vi "regser Main.vi"() -> ()   [LabVIEW 2015]
doc: "This template is for the Queued Message Handler design pattern.\n\nThe Event Handling Loop generates messages based on user interface actions.\n\nThe Message Handling Loop processes messages generated by the Event Handling Loop, or by other messages. The messages are string values, so new messages can be added easily to the Message Cases case structure in the Message Handling Loop. Each message cluster can also provide an optional value for Message Data, which is a variant that can be converted to whatever message-specific data is required."
uses:
  Type Definitions/status_LED.ctl
  controls/regser UI Data.ctl
  init_config/typedef/init_config_data.ctl
  controls/config Data.ctl
  support/Message Queue/Enqueue Message (Single).vi
  <vilib>/Utility/error.llb/Error Cluster From Error Code.vi
  <vilib>/ErrorRing/Error Ring.xnode
  support/Message Queue/regser Message Queue.lvlib
  support/User Event - Stop/regser User Event - Stop.lvlib
panel:
  out "sw ver":string
  out "Enpoint":string
  in  "Exit Button":bool
  out "Target":dbl caption="Tgt"
  out "No. rej":i32
  out "Rejected":i32(slide) caption="Rejected test logs" scale=0.0..20.0
  out "No. pend":i32
  out "Pending":i32(slide) caption="Pending test logs" scale=0.0..20.0
  out "No. acc":i32
  out "Accepted":i32(slide) caption="Accepted test logs" scale=0.0..1000.0
  out "ext.":string caption="searching for"
  in  "Stop Button":bool
  in  "Start Button":bool
  out "Messages":string
  out "status":T1
  out "Elapsed time":dbl format="%.1f"
  out "Run":bool
  out "Display <Replace Me>":string
  # "QMH based"
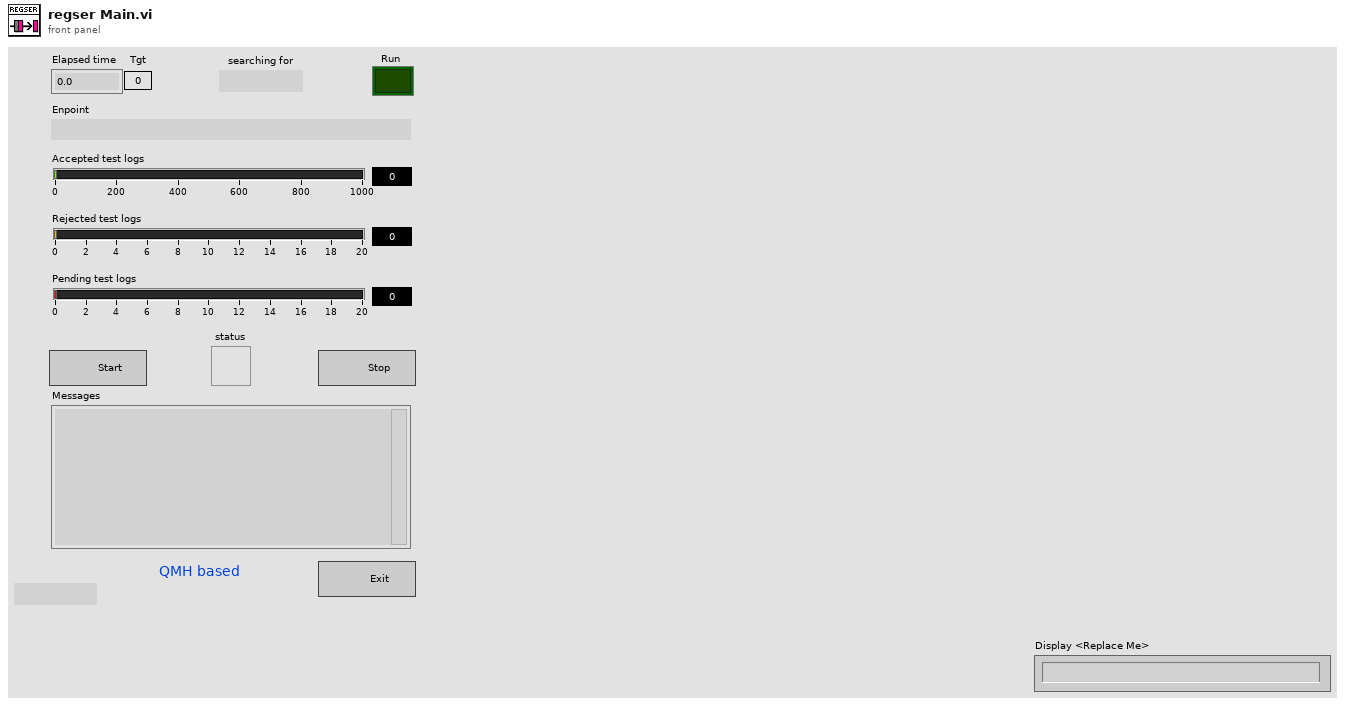
[diagram p1: front panel]
types:
  T1 = typedef "status_LED.ctl" = bool
  T2 = typedef "config Data.ctl" = cluster{"Boolean <Replace Me>":bool, "String <Replace Me>":string, "Numeric <Replace Me>":dbl, "http timeout":cluster{"get_timeout":i32, "post_timeout":i32}}
  T3 = typedef "regser UI Data.ctl" = cluster{"Boolean <Replace Me>":bool, "String <Replace Me>":string, "Numeric <Replace Me>":dbl, "Do Something Ref":refnum<vi>, "Do Something Else Ref":refnum<vi>, "Data Display Ref":refnum<vi>, "Exit Button Ref":refnum<vi>, "Cfg Data":T4, "Folder Path out":path, "All Files in Dir":path[], "No. of Files":i32, "Err Msg":string, "Err status":bool}
  T4 = typedef "init_config_data.ctl" = cluster{"http timeout":cluster{"get_timeout":i32, "post_timeout":i32}, "folders":cluster{"test_log_base_path":string, "accepted_folder_name":string, "rejected_folder_name":string}, "end_point":string, "file_ext":string, "holding time":dbl}
  T5 = typedef "regser Message Queue.lvlib/All Message Queues.ctl" = cluster{"UI":refnum<queue>, "CNFG":refnum<queue>}
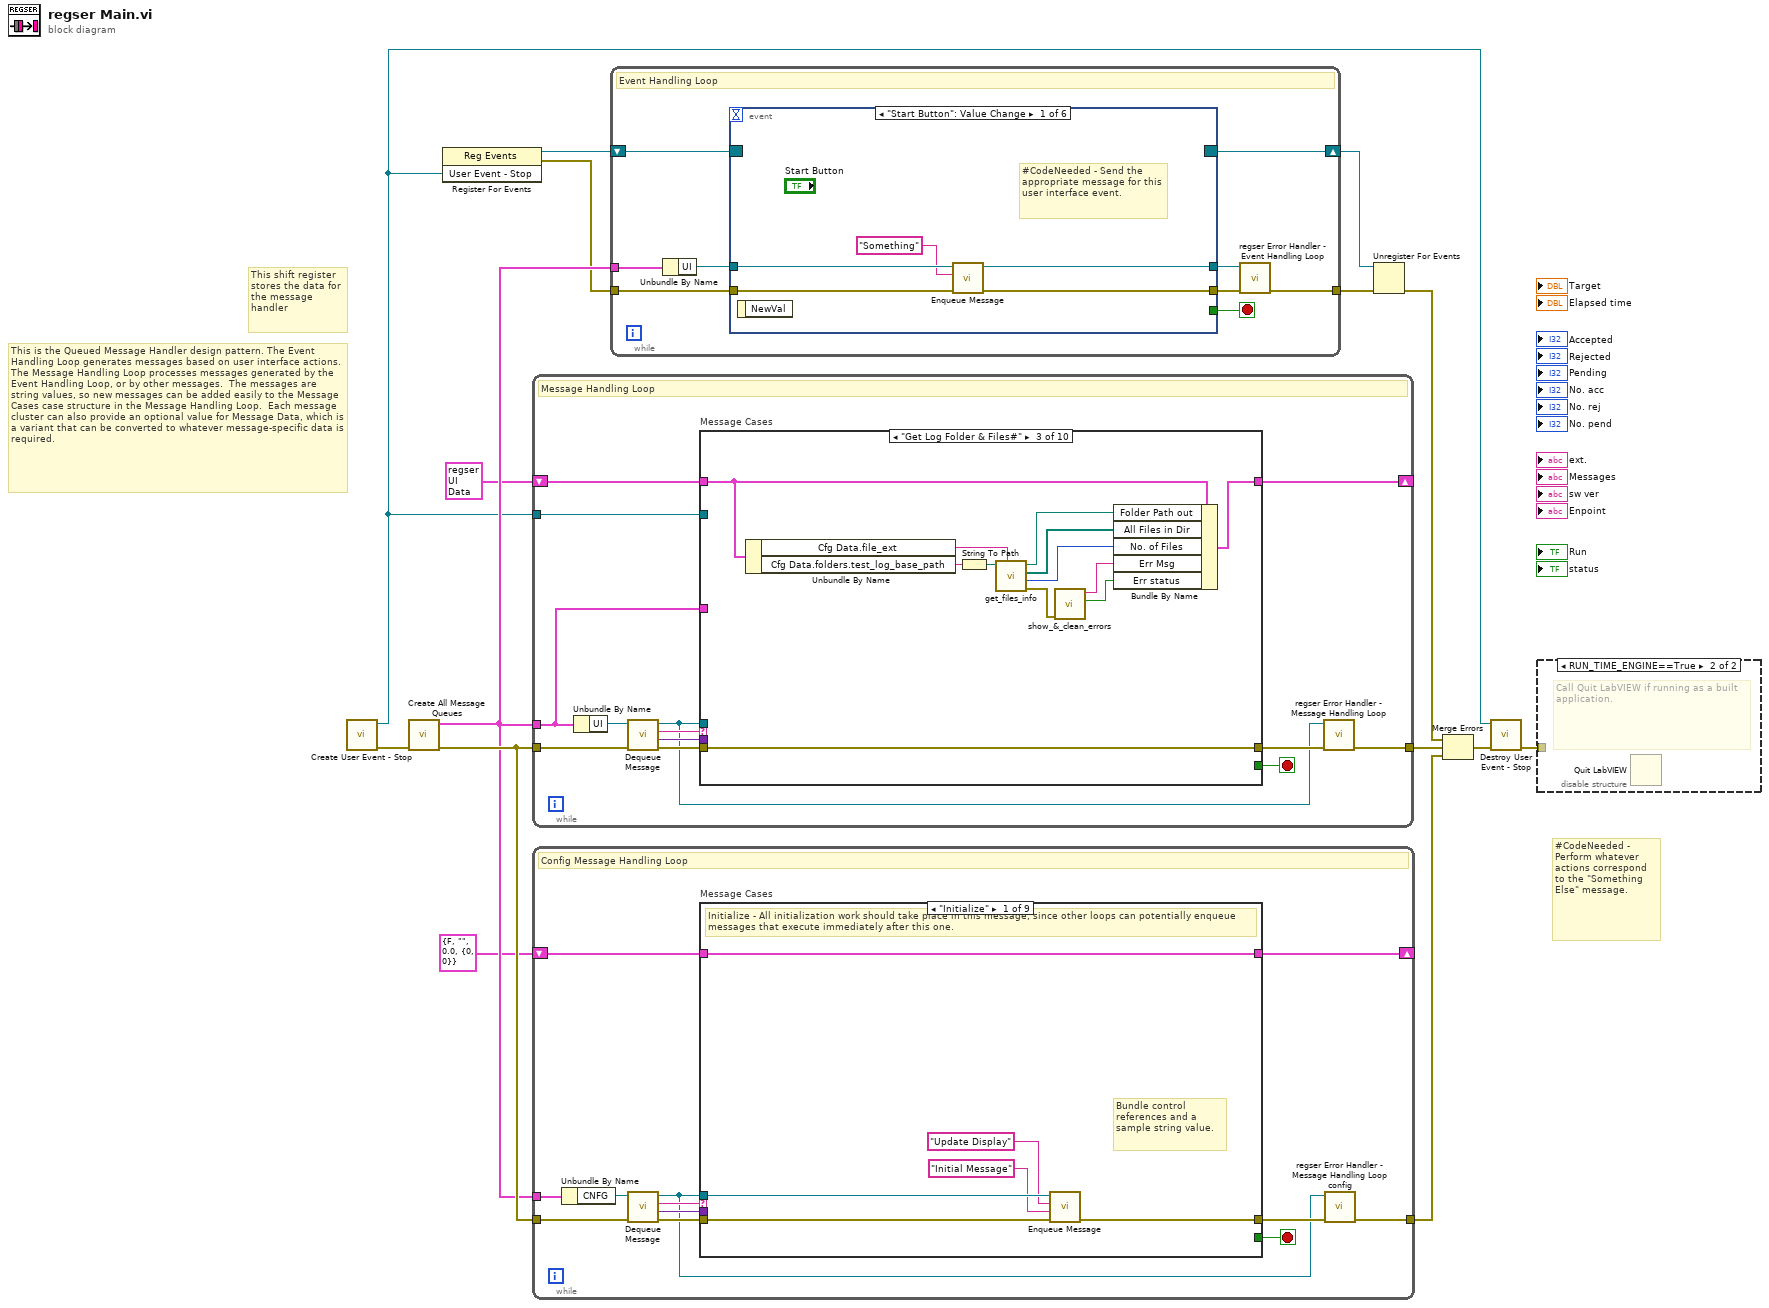
[diagram p0: block diagram]
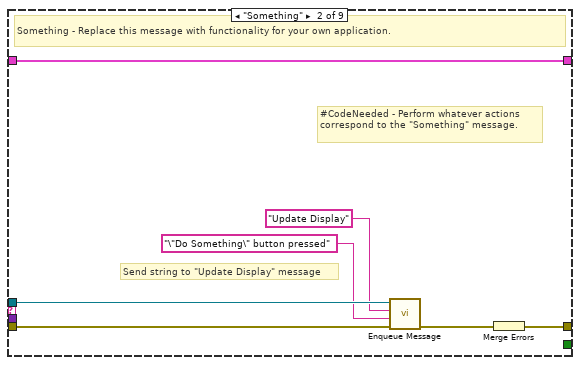
[diagram p2: hidden frame]
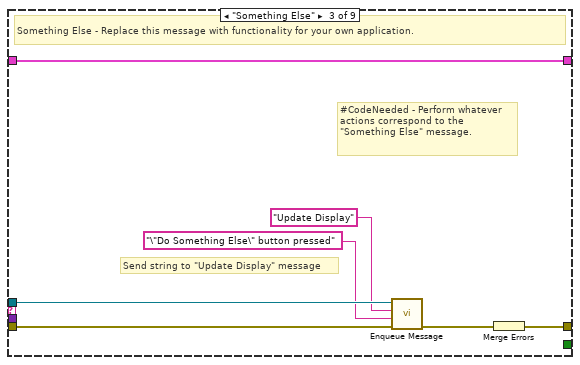
[diagram p3: hidden frame]
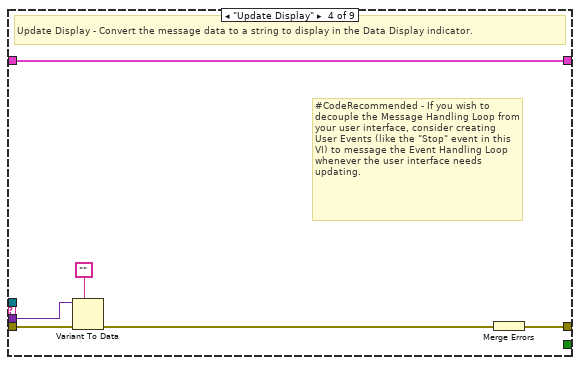
[diagram p4: hidden frame]
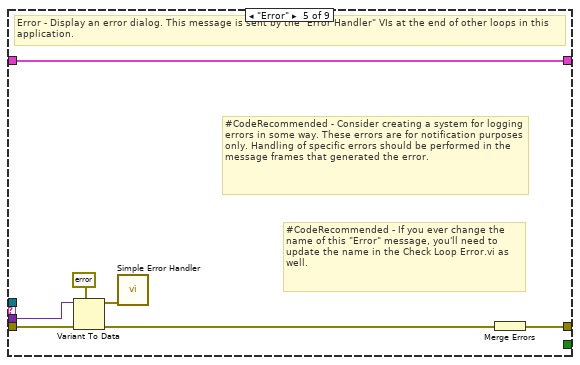
[diagram p5: hidden frame]
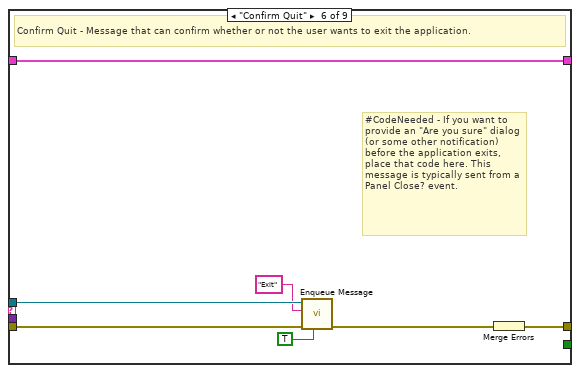
[diagram p6: hidden frame]
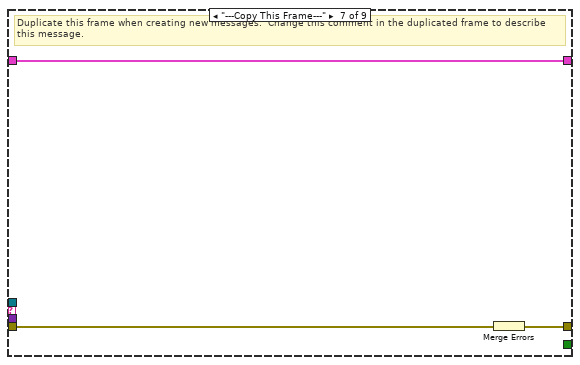
[diagram p7: hidden frame]
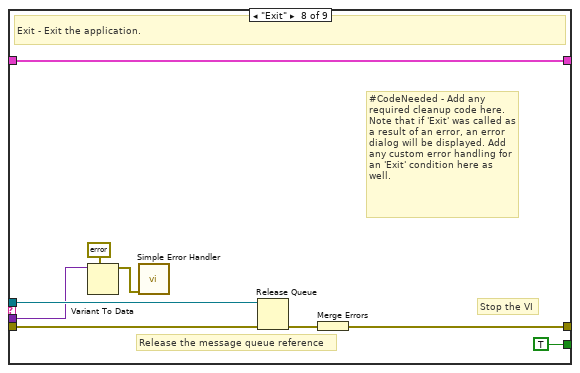
[diagram p8: hidden frame]
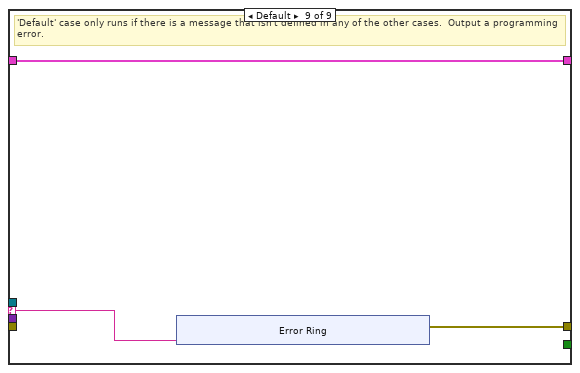
[diagram p9: hidden frame]
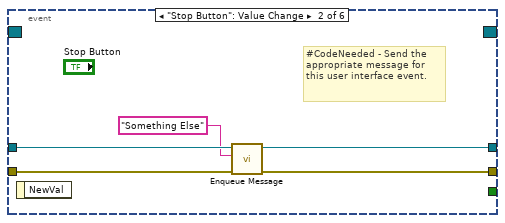
[diagram p11: hidden frame]
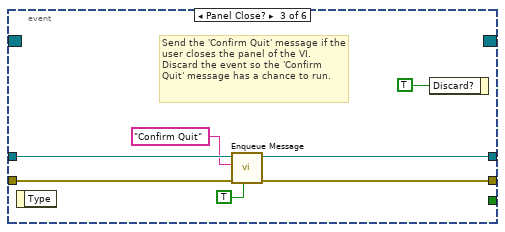
[diagram p12: hidden frame]
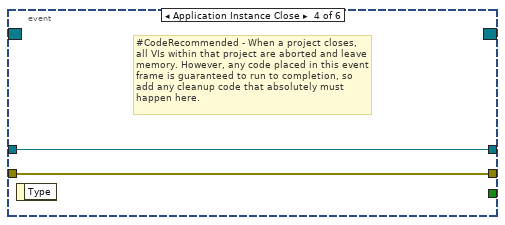
[diagram p13: hidden frame]
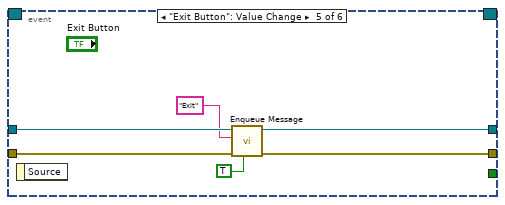
[diagram p14: hidden frame]
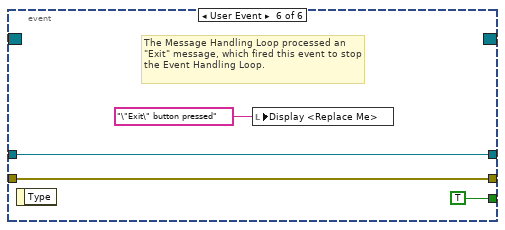
[diagram p15: hidden frame]
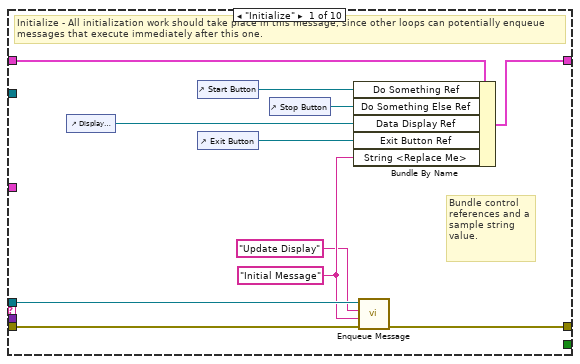
[diagram p16: hidden frame]
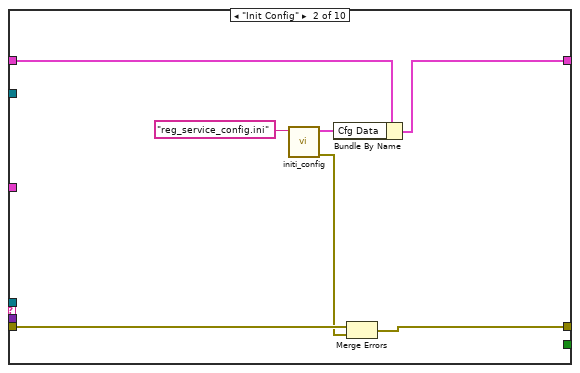
[diagram p17: hidden frame]
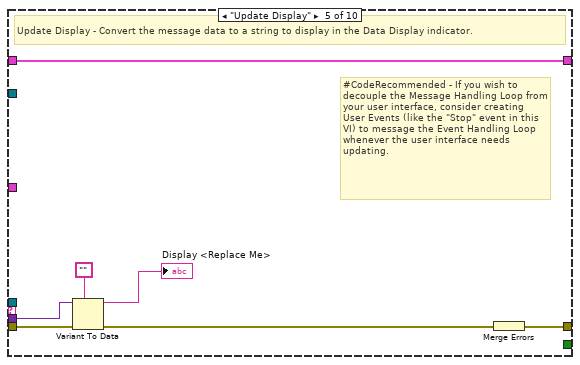
[diagram p19: hidden frame]
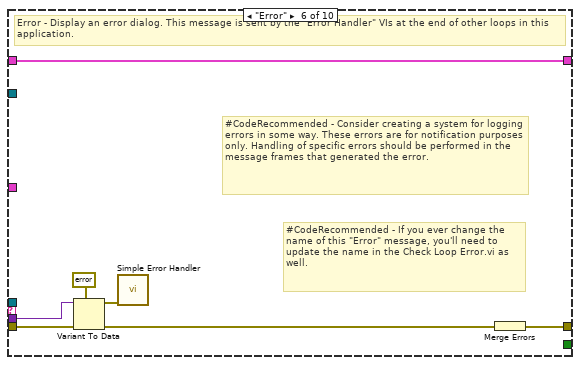
[diagram p20: hidden frame]
diagram:
  # "#CodeNeeded - Perform whatever actions correspond to the \"Something Else\" message."
  # "This is the Queued Message Handler design pattern. The Event Handling Loop generates messages based on user interface actions. The Message Handling Loop processes messages generated by the Event Handling Loop, or by other messages.  The messages are string values, so new messages can be added easily to the Message Cases case structure in the Message Handling Loop.  Each message cluster can also provide an optional value for Message Data, which is a variant that can be converted to whatever message-specific data is required."
  # "This shift register stores the data for the message handler"
  n1 = call "Create User Event - Stop.vi"() -> ("error out"=w12:errorcluster, "User Event - Stop"=w4:refnum<user-event>)  [unwired: 10 in]
  n2 = call "Create All Message Queues.vi"("error in (no error)"=w12) -> ("error out"=w15:errorcluster, "Message Queues out"=w14:T5)  [unwired: 9 in]
  n3 = register-events(w4) -> (reference out=w5:refnum<event-registration>, error out=w1:errorcluster)  [unwired: 2 in]
  n4 = while {
    shift-right: [w27] -> _
    shift-left: T3 {"Boolean <Replace Me>"=FALSE, "String <Replace Me>"="", "Numeric <Replace Me>"=0.0, "Do Something Ref"=refnum, "Do Something Else Ref"=refnum, "Data Display Ref"=refnum, "Exit Button Ref"=refnum, "Cfg Data"={"http timeout"={"get_timeout"=0, "post_timeout"=0}, "folders"={"test_log_base_path"="", "accepted_folder_name"="", "rejected_folder_name"=""}, "end_point"="", "file_ext"="", "holding time"=0.0}, "Folder Path out"=path "", "All Files in Dir"=[], "No. of Files"=0, "Err Msg"="", "Err status"=FALSE} ("Data Cluster") -> [w28]
    tunnel: w4 -> [w25]
    tunnel: w15 -> [w24]
    tunnel: [w20] -> w13
    tunnel: w14 -> [w16]
    stop <- w26 stop-if-true
    # "Message Handling Loop"
    n5 = Unbundle By Name(w16) -> ("UI"=w17:refnum<queue>)
    n6 = call "Dequeue Message.vi"("error in (no error)"=w24, "Message Queue"=w17) -> ("error out"=w23:errorcluster, "Message Data"=w21:variant, "Message"=w22:string, "dup Message Queue"=w18:refnum<queue>)  [unwired: 6 in]
    n7 = case "Message Cases" shown="\"Get Log Folder & Files#\"" w22 {
      selector: w22 -> [_ _ _ _ _ _ _ _ _ w101]
      tunnel: w18 -> [w31 _ _ _ _ _ w77 _ w100 _]
      tunnel: w23 -> [w38 w46 w58 w60 w65 w74 w81 w84 w93 _]
      tunnel: [w39 w45 w58 w60 w66 w68 w79 w82 w96 w102] -> w19
      tunnel: w28 -> [w37 w43 w53 w59 w67 w73 w80 w83 w99 w103]
      tunnel: [w36 w41 w52 w59 w67 w73 w80 w83 w99 w103] -> w27
      tunnel: [_ _ _ _ _ _ _ _ TRUE _] -> w26
      tunnel: w21 -> [_ _ _ _ w64 w72 _ _ w90 _]
      tunnel: w25 -> [_ _ _ _ _ _ _ _ w95 _]
      tunnel: w16 -> [_ _ _ _ _ _ _ _ w86 _]
      frame "Initialize" {
        w30 = "Initial Message" ("Initial Message")
        # "Bundle control references and a sample string value."
        # "Initialize - All initialization work should take place in this message, since other loops can potentially enqueue messages that execute immediately after this one."
        n8 = control-ref of="Display <Replace Me>"() -> (w33:refnum<vi>)
        n9 = control-ref of="Start Button"() -> (w35:refnum<vi>)
        n10 = control-ref of="Exit Button"() -> (w32:refnum<vi>)
        n11 = control-ref of="Stop Button"() -> (w34:refnum<vi>)
        n12 = Bundle By Name(cluster=w37, "Do Something Ref"=w35, "Do Something Else Ref"=w34, "Data Display Ref"=w33, "Exit Button Ref"=w32, "String <Replace Me>"=w30) -> (w36:T3)
        n13 = call-poly "Enqueue Message.vi"("error in (no error)"=w38, "Message Data"=w30, "Message"="Update Display", "Message Queue"=w31) -> ("error out"=w39:errorcluster)  [unwired: 6 in, 1 out]
      }
      frame "Init Config" {
        n14 = call "initi_config.vi"("config_file_name"="reg_service_config.ini") -> ("error out"=w44:errorcluster, "Cfg Data"=w42:T4)  [unwired: 9 in]
        n15 = Bundle By Name(cluster=w43, "Cfg Data"=w42) -> (w41:T3)
        n16 = Merge Errors(w46, w44) -> (w45:errorcluster)
      }
      frame "Get Log Folder & Files#" {
        n17 = Unbundle By Name(w53) -> ("Cfg Data.file_ext"=w54:string, "Cfg Data.folders.test_log_base_path"=w57:string)
        n18 = String To Path(string=w57) -> (path=w56:path)
        n19 = call "get_files_info.vi"("pattern"=w54, "Folder path in"=w56) -> ("error out"=w55:errorcluster, "Number of Files"=w49:i32, "All Files in Dir"=w50:path[], "Folder Path out"=w51:path)  [unwired: 6 in]
        n20 = call "show_&_clean_errors.vi"("error in (no error)"=w55) -> ("status"=w47:bool, "message out"=w48:string)  [unwired: 7 in, 2 out]
        n21 = Bundle By Name(cluster=w53, "Folder Path out"=w51, "All Files in Dir"=w50, "No. of Files"=w49, "Err Msg"=w48, "Err status"=w47) -> (w52:T3)
      }
      frame "Idle" {
      }
      frame "Update Display" {
        # "#CodeRecommended - If you wish to decouple the Message Handling Loop from your user interface, consider creating User Events (like the \"Stop\" event in this VI) to message the Event Handling Loop whenever the user interface needs updating."
        # "Update Display - Convert the message data to a string to display in the Data Display indicator."
        n22 = Variant To Data(error in=w65, type="", Variant=w64) -> (data=→"Display <Replace Me>":string, error out=w62:errorcluster)
        n23 = Merge Errors(w62) -> (w66:errorcluster)
      }
      frame "Error" {
        # "#CodeRecommended - If you ever change the name of this \"Error\" message, you'll need to update the name in the Check Loop Error.vi as well."
        # "#CodeRecommended - Consider creating a system for logging errors in some way. These errors are for notification purposes only. Handling of specific errors should be performed in the message frames that generated the error."
        # "Error - Display an error dialog. This message is sent by the \"Error Handler\" VIs at the end of other loops in this application."
        n24 = Variant To Data(error in=w74, type=errorcluster {"status"=FALSE, "code"=0, "source"=""} ("error constant"), Variant=w72) -> (data=w70:errorcluster, error out=w69:errorcluster)
        n25 = call <vilib>:"Simple Error Handler.vi"("error in (no error)"=w70) -> ()  [unwired: 4 in, 5 out]
        n26 = Merge Errors(w69) -> (w68:errorcluster)
      }
      frame "Confirm Quit" {
        # "#CodeNeeded - If you want to provide an \"Are you sure\" dialog (or some other notification) before the application exits, place that code here. This message is typically sent from a Panel Close? event."
        # "Confirm Quit - Message that can confirm whether or not the user wants to exit the application."
        n27 = call-poly "Enqueue Message.vi"("Priority Message? (F)"=TRUE, "error in (no error)"=w81, "Message"="Exit", "Message Queue"=w77) -> ("error out"=w78:errorcluster)  [unwired: 6 in, 1 out]
        n28 = Merge Errors(w78) -> (w79:errorcluster)
      }
      frame "---Copy This Frame---" {
        # "Duplicate this frame when creating new messages.  Change this comment in the duplicated frame to describe this message."
        n29 = Merge Errors(w84) -> (w82:errorcluster)
      }
      frame "Exit" {
        # "Stop the VI"
        # "Release the message queue reference"
        # "#CodeNeeded - Add any required cleanup code here. Note that if 'Exit' was called as a result of an error, an error dialog will be displayed. Add any custom error handling for an 'Exit' condition here as well."
        # "Exit - Exit the application."
        n30 = Variant To Data(type=errorcluster {"status"=FALSE, "code"=0, "source"=""} ("error constant"), Variant=w90) -> (data=w91:errorcluster)  [unwired: 1 in, 1 out]
        n31 = call <vilib>:"Simple Error Handler.vi"("error in (no error)"=w91) -> ()  [unwired: 4 in, 5 out]
        n32 = Unbundle By Name(w86) -> ("CNFG"=w88:refnum<queue>)
        n33 = Release Queue(queue=w100, error in (no error)=w93) -> (error out=w97:errorcluster)  [unwired: 1 in, 2 out]
        n34 = call-poly "Enqueue Message.vi"("Priority Message? (F)"=TRUE, "Message"="Exit", "Message Queue"=w88) -> ("error out"=w85:errorcluster)  [unwired: 7 in, 1 out]
        n35 = call "Fire User Event - Stop.vi"("User Event - Stop"=w95) -> ("error out"=w94:errorcluster)  [unwired: 10 in]
        n36 = Merge Errors(w94, w85, w97) -> (w96:errorcluster)
      }
      frame Default {
        # "'Default' case only runs if there is a message that isn't defined in any of the other cases.  Output a programming error."
        n37 = xnode "Error Ring"("parameter 0"=w101) -> ("error out"=w102:errorcluster)
      }
    }
    n38 = call "regser Error Handler - Message Handling Loop.vi"("error in (no error)"=w19, "Message Queue"=w18) -> ("dup error in"=w20:errorcluster)  [unwired: 8 in, 1 out]
  }
  n39 = while {
    shift-right: [w121] -> _
    shift-left: T2 {"Boolean <Replace Me>"=FALSE, "String <Replace Me>"="", "Numeric <Replace Me>"=0.0, "http timeout"={"get_timeout"=0, "post_timeout"=0}} ("Data Cluster") -> [w122]
    tunnel: w15 -> [w119]
    tunnel: [w115] -> w2
    tunnel: w14 -> [w111]
    stop <- w120 stop-if-true
    # "Config Message Handling Loop"
    n40 = Unbundle By Name(w111) -> ("CNFG"=w112:refnum<queue>)
    n41 = call "Dequeue Message.vi"("error in (no error)"=w119, "Message Queue"=w112) -> ("error out"=w118:errorcluster, "Message Data"=w116:variant, "Message"=w117:string, "dup Message Queue"=w113:refnum<queue>)  [unwired: 6 in]
    n42 = case "Message Cases" shown="\"Initialize\"" w117 {
      selector: w117 -> [_ _ _ _ _ _ _ _ w175]
      tunnel: w113 -> [w126 w131 w138 _ _ w158 _ w174 _]
      tunnel: w118 -> [w127 w133 w140 w146 w155 w162 w165 w169 _]
      tunnel: [w128 w134 w141 w147 w149 w160 w163 w170 w176] -> w114
      tunnel: w122 -> [w123 w135 w142 w148 w154 w161 w164 w173 w177]
      tunnel: [w123 w135 w142 w148 w154 w161 w164 w173 w177] -> w121
      tunnel: [_ _ _ _ _ _ _ TRUE _] -> w120
      tunnel: w116 -> [_ _ _ w145 w153 _ _ w166 _]
      frame "Initialize" {
        # "Bundle control references and a sample string value."
        # "Initialize - All initialization work should take place in this message, since other loops can potentially enqueue messages that execute immediately after this one."
        n43 = call-poly "Enqueue Message.vi"("error in (no error)"=w127, "Message Data"="Initial Message" ("Initial Message"), "Message"="Update Display", "Message Queue"=w126) -> ("error out"=w128:errorcluster)  [unwired: 6 in, 1 out]
      }
      frame "Something" {
        # "Send string to \"Update Display\" message"
        # "#CodeNeeded - Perform whatever actions correspond to the \"Something\" message."
        # "Something - Replace this message with functionality for your own application."
        n44 = call-poly "Enqueue Message.vi"("error in (no error)"=w133, "Message Data"="\"Do Something\" button pressed" ("\"Do Something\" button pressed"), "Message"="Update Display", "Message Queue"=w131) -> ("error out"=w132:errorcluster)  [unwired: 6 in, 1 out]
        n45 = Merge Errors(w132) -> (w134:errorcluster)
      }
      frame "Something Else" {
        # "Send string to \"Update Display\" message"
        # "#CodeNeeded - Perform whatever actions correspond to the \"Something Else\" message."
        # "Something Else - Replace this message with functionality for your own application."
        n46 = call-poly "Enqueue Message.vi"("error in (no error)"=w140, "Message Data"="\"Do Something Else\" button pressed" ("\"Do Something Else\" button pressed"), "Message"="Update Display", "Message Queue"=w138) -> ("error out"=w139:errorcluster)  [unwired: 6 in, 1 out]
        n47 = Merge Errors(w139) -> (w141:errorcluster)
      }
      frame "Update Display" {
        # "#CodeRecommended - If you wish to decouple the Message Handling Loop from your user interface, consider creating User Events (like the \"Stop\" event in this VI) to message the Event Handling Loop whenever the user interface needs updating."
        # "Update Display - Convert the message data to a string to display in the Data Display indicator."
        n48 = Variant To Data(error in=w146, type="", Variant=w145) -> (error out=w143:errorcluster)  [unwired: 1 out]
        n49 = Merge Errors(w143) -> (w147:errorcluster)
      }
      frame "Error" {
        # "#CodeRecommended - If you ever change the name of this \"Error\" message, you'll need to update the name in the Check Loop Error.vi as well."
        # "#CodeRecommended - Consider creating a system for logging errors in some way. These errors are for notification purposes only. Handling of specific errors should be performed in the message frames that generated the error."
        # "Error - Display an error dialog. This message is sent by the \"Error Handler\" VIs at the end of other loops in this application."
        n50 = Variant To Data(error in=w155, type=errorcluster {"status"=FALSE, "code"=0, "source"=""} ("error constant"), Variant=w153) -> (data=w151:errorcluster, error out=w150:errorcluster)
        n51 = call <vilib>:"Simple Error Handler.vi"("error in (no error)"=w151) -> ()  [unwired: 4 in, 5 out]
        n52 = Merge Errors(w150) -> (w149:errorcluster)
      }
      frame "Confirm Quit" {
        # "#CodeNeeded - If you want to provide an \"Are you sure\" dialog (or some other notification) before the application exits, place that code here. This message is typically sent from a Panel Close? event."
        # "Confirm Quit - Message that can confirm whether or not the user wants to exit the application."
        n53 = call-poly "Enqueue Message.vi"("Priority Message? (F)"=TRUE, "error in (no error)"=w162, "Message"="Exit", "Message Queue"=w158) -> ("error out"=w159:errorcluster)  [unwired: 6 in, 1 out]
        n54 = Merge Errors(w159) -> (w160:errorcluster)
      }
      frame "---Copy This Frame---" {
        # "Duplicate this frame when creating new messages.  Change this comment in the duplicated frame to describe this message."
        n55 = Merge Errors(w165) -> (w163:errorcluster)
      }
      frame "Exit" {
        # "Stop the VI"
        # "Release the message queue reference"
        # "#CodeNeeded - Add any required cleanup code here. Note that if 'Exit' was called as a result of an error, an error dialog will be displayed. Add any custom error handling for an 'Exit' condition here as well."
        # "Exit - Exit the application."
        n56 = Variant To Data(type=errorcluster {"status"=FALSE, "code"=0, "source"=""} ("error constant"), Variant=w166) -> (data=w167:errorcluster)  [unwired: 1 in, 1 out]
        n57 = call <vilib>:"Simple Error Handler.vi"("error in (no error)"=w167) -> ()  [unwired: 4 in, 5 out]
        n58 = Release Queue(queue=w174, error in (no error)=w169) -> (error out=w171:errorcluster)  [unwired: 1 in, 2 out]
        n59 = Merge Errors(w171) -> (w170:errorcluster)
      }
      frame Default {
        # "'Default' case only runs if there is a message that isn't defined in any of the other cases.  Output a programming error."
        n60 = xnode "Error Ring"("parameter 0"=w175) -> ("error out"=w176:errorcluster)
      }
    }
    n61 = call "regser Error Handler - Message Handling Loop config.vi"("error in (no error)"=w114, "Message Queue"=w113) -> ("dup error in"=w115:errorcluster)  [unwired: 8 in, 1 out]
  }
  n62 = while {
    shift-right: [w192] -> w9
    shift-left: w5 -> [w193]
    tunnel: [w188] -> w6
    tunnel: w14 -> [w187]
    tunnel: w1 -> [w185]
    stop <- w190 stop-if-true
    # "Event Handling Loop"
    n63 = Unbundle By Name(w187) -> ("UI"=w186:refnum<queue>)
    n64 = event shown="[0] \"Start Button\": Value Change" {
      selector: w193 -> [_ _ _ _ _ _]
      dyn-events: [_ _ _ _ _ _] -> w192
      timeout: _ -> [_ _ _ _ _ _]
      tunnel: [_ _ _ _ _ TRUE ("Discard?")] -> w190
      tunnel: w186 -> [w198 w203 w209 w212 w218 w222]
      tunnel: [w195 w200 w208 w211 w217 w219] -> w191
      tunnel: [w197 w202 w207 w212 w216 w222] -> w189
      tunnel: w185 -> [w194 w199 w204 w211 w213 w219]
      event "Start Button": Value Change {
        # "#CodeNeeded - Send the appropriate message for this user interface event."
        n65 = event-data() -> ()  [unwired: 1 in, 1 out]
        n66 = call-poly "Enqueue Message.vi"("error in (no error)"=w194, "Message"="Something", "Message Queue"=w198) -> ("error out"=w195:errorcluster, "dup Message Queue"=w197:refnum<queue>)  [unwired: 7 in]
      }
      event "Stop Button": Value Change {
        # "#CodeNeeded - Send the appropriate message for this user interface event."
        n67 = event-data() -> ()  [unwired: 1 in, 1 out]
        n68 = call-poly "Enqueue Message.vi"("error in (no error)"=w199, "Message"="Something Else", "Message Queue"=w203) -> ("error out"=w200:errorcluster, "dup Message Queue"=w202:refnum<queue>)  [unwired: 7 in]
      }
      event Panel Close? {
        # "Send the 'Confirm Quit' message if the user closes the panel of the VI. Discard the event so the 'Confirm Quit' message has a chance to run."
        n69 = event-data() -> ()  [unwired: 1 in, 1 out]
        n70 = call-poly "Enqueue Message.vi"("Priority Message? (F)"=TRUE, "error in (no error)"=w204, "Message"="Confirm Quit", "Message Queue"=w209) -> ("error out"=w208:errorcluster, "dup Message Queue"=w207:refnum<queue>)  [unwired: 6 in]
        n71 = event-data("Discard?"=TRUE) -> ()  [unwired: 1 in, 1 out]
      }
      event Application Instance Close {
        # "#CodeRecommended - When a project closes, all VIs within that project are aborted and leave memory. However, any code placed in this event frame is guaranteed to run to completion, so add any cleanup code that absolutely must happen here."
        n72 = event-data() -> ()  [unwired: 1 in, 1 out]
      }
      event "Exit Button": Value Change {
        n73 = event-data() -> ()  [unwired: 1 in, 1 out]
        n74 = call-poly "Enqueue Message.vi"("Priority Message? (F)"=TRUE, "error in (no error)"=w213, "Message"="Exit", "Message Queue"=w218) -> ("error out"=w217:errorcluster, "dup Message Queue"=w216:refnum<queue>)  [unwired: 6 in]
      }
      event User Event {
        # "The Message Handling Loop processed an \"Exit\" message, which fired this event to stop the Event Handling Loop."
        n75 = event-data() -> ()  [unwired: 1 in, 1 out]
        n76 = local write "Display <Replace Me>"("\"Exit\" button pressed" ("VI Stopped")) -> ()
      }
    }
    n77 = call "regser Error Handler - Event Handling Loop.vi"("error in (no error)"=w191, "Message Queue"=w189) -> ("dup error in"=w188:errorcluster)  [unwired: 8 in, 1 out]
  }
  n78 = Unregister For Events(event registration refnum=w9, error in=w6) -> (error out=w10:errorcluster)
  n79 = Merge Errors(w10, w13, w2) -> (w11:errorcluster)
  n80 = call "Destroy User Event - Stop.vi"("error in (no error)"=w11, "User Event - Stop"=w4) -> ("error out"=w7:errorcluster)  [unwired: 9 in]
  n81 = disable-structure shown="RUN_TIME_ENGINE==True" {
    disable-tunnel: w7 -> [_ _]
    frame condition #0 (active) {
    }
    frame condition #1 {
      # "Call Quit LabVIEW if running as a built application."
      n82 = Quit LabVIEW() -> ()  [unwired: 1 in]
    }
  }
